vi "Fetch (Unscaled Int16).vi"(0 "VISA resource name":refnum<visa-resource-name>, 1 "Segment Index (0)":i32 format="%.0g", 5 "Measurement Source (1: Channel 1)":i32(ring)=1 items=["Channel 1"=1, "Channel 2"=2, "Channel 3"=3, "Channel 4"=4, "Function 1"=5, "Function 2"=6, "Function 3"=7, "Function 4"=8, "Memory 1"=9, "Memory 2"=10, "Memory 3"=11, "Memory 4"=12], 7 "Number of Samples (1000)":i32=10000 caption="Number of Samples (10000)", 9 "Maximum Time (10000ms)":u32=10000, 11 "error in (no error)":errorcluster, 12 "Offset (0)":i32) -> (4 "VISA resource name out":refnum<visa-resource-name>, 6 "Waveform Information":T1, 8 "Waveform Data":i16[](array[numeric]), 15 "error out":errorcluster)   [LabVIEW 2020, in "Agilent 90000 Series.lvlib"]
doc: "Fetches the unscaled raw word data from instrument. Use this VI under word data format configuration."
uses:
  Agilent 90000 Series.lvlib
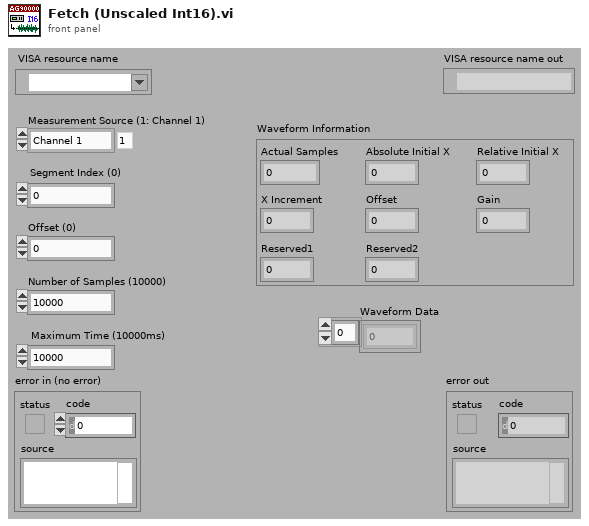
[diagram p1: front panel]
types:
  T1 = cluster{"Actual Samples":i32, "Absolute Initial X":dbl, "Relative Initial X":dbl, "X Increment":dbl, "Offset":dbl, "Gain":dbl, "Reserved1":dbl, "Reserved2":dbl}
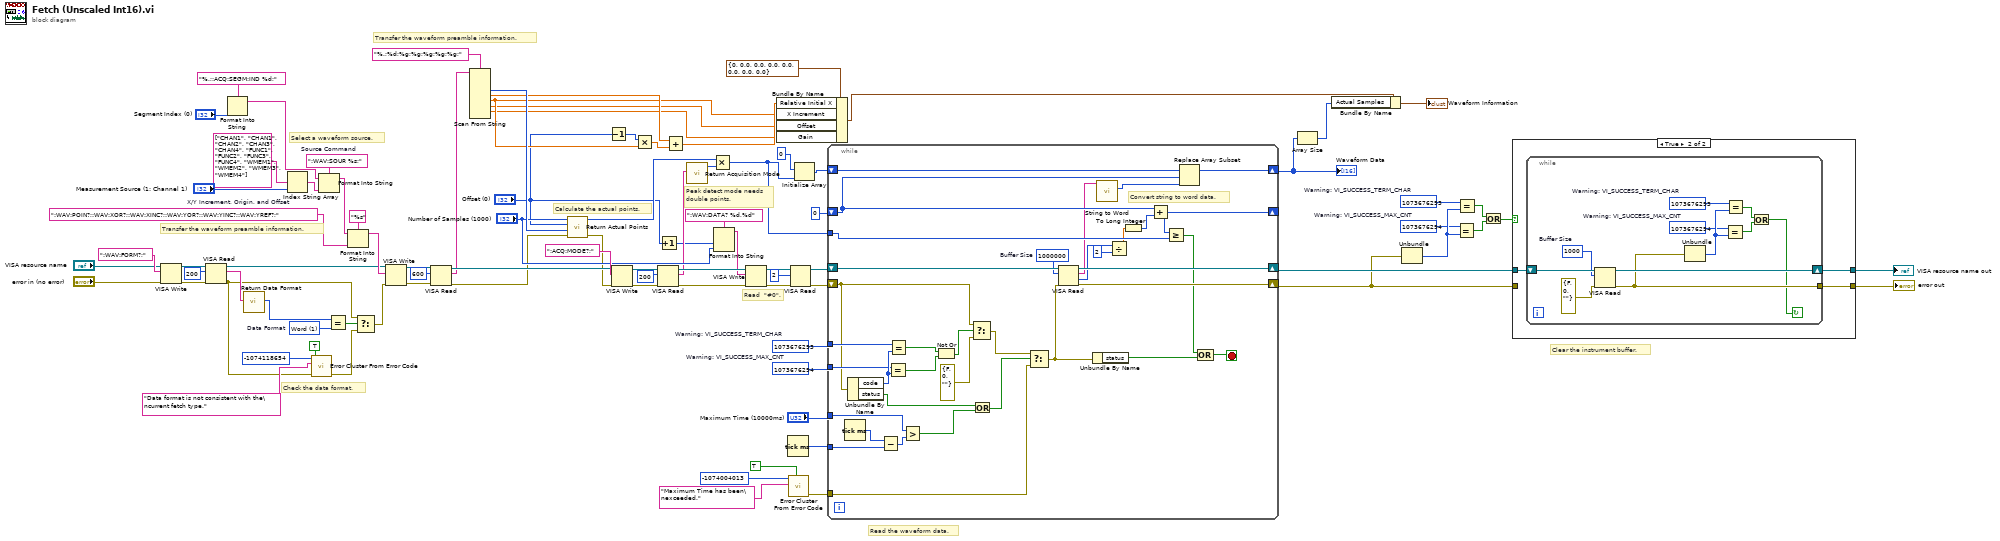
[diagram p0: block diagram]
diagram:
  w18 = u16 1 items=["Byte", "Word", "Others"]  # Data Format
  w74 = 1073676294  # Warning: VI_SUCCESS_MAX_CNT
  w73 = 1073676293  # Warning: VI_SUCCESS_TERM_CHAR
  w67 = 1073676294  # Warning: VI_SUCCESS_MAX_CNT
  w66 = 1073676293  # Warning: VI_SUCCESS_TERM_CHAR
  w87 = ":WAV:SOUR %s;"  # Source Command
  w81 = ":WAV:POIN?;:WAV:XOR?;:WAV:XINC?;:WAV:YOR?;:WAV:YINC?;:WAV:YREF?;"  # X/Y Increment, Origin, and Offset
  # "Transfer the waveform preamble information."
  # "Peak detect mode needs\ndouble points."
  # "Calculate the actual points."
  # "Check the data format."
  # "Read  \"#0\"."
  # "Clear the instrument buffer."
  # "Read the waveform data."
  # "Select a waveform source."
  # "Transfer the waveform preamble information."
  n1 = VISA Write(VISA resource name="VISA resource name", write buffer=":WAV:FORM?;", error in (no error)="error in (no error)") -> (VISA resource name out=w35:refnum<visa-resource-name>, error out=w34:errorcluster)  [unwired: 1 out]
  n2 = VISA Read(VISA resource name=w35, byte count=u32 200, error in (no error)=w34) -> (VISA resource name out=w31:refnum<visa-resource-name>, read buffer=w28:string, error out=w5:errorcluster)  [unwired: 1 out]
  n3 = Format Into String(format string="%.;:ACQ:SEGM:IND %d;", "Segment Index (0)") -> (resulting string=w2:string)  [unwired: 2 in, 1 out]
  n4 = call "Return Data Format.vi"("String In"=w28) -> ("Data Format"=w25:u16)  [unwired: 1 in, 9 out]
  n5 = Index String Array(1:"Measurement Source (1: Channel 1)", 2:string[] ["CHAN1", "CHAN1", "CHAN2", "CHAN3", "CHAN4", "FUNC1", "FUNC2", "FUNC3", "FUNC4", "WMEM1", "WMEM2", "WMEM3", "WMEM4"] ("subarray 2")) -> (0:w82:string)  [unwired: 1 out]
  n6 = call <vilib>:"Error Cluster From Error Code.vi"("show call chain? (False)"=TRUE, "error in (no error)"=w5, "error message (\"\")"="Data format is not consistent with the\ncurrent fetch type." ("error message (\"\")"), "error code (0)"=-1074118654) -> ("error out"=w19:errorcluster)  [unwired: 5 out]
  n7 = Format Into String(format string=w87, initial string=w2, w82) -> (resulting string=w85:string)  [unwired: 1 in, 1 out]
  n8 = Equal?(x=w25, y=w18) -> (x = y?=w24:bool)
  n9 = Format Into String(format string="%s", initial string=w85, w81) -> (resulting string=w84:string)  [unwired: 1 in, 1 out]
  n10 = Select(t=w5, s=w24, f=w19) -> (s? t:f=w23:errorcluster)
  n11 = VISA Write(VISA resource name=w31, write buffer=w84, error in (no error)=w23) -> (VISA resource name out=w90:refnum<visa-resource-name>, error out=w89:errorcluster)  [unwired: 1 out]
  n12 = VISA Read(VISA resource name=w90, byte count=u32 600, error in (no error)=w89) -> (VISA resource name out=w60:refnum<visa-resource-name>, read buffer=w46:string, error out=w9:errorcluster)  [unwired: 1 out]
  n13 = Scan From String(format string="%.;%d;%g;%g;%g;%g;%g;", input string=w46) -> (output 1=w47:i32, output 2=w45:dbl, output 3=w44:dbl, output 4=w13:dbl, output 5=w7:dbl)  [unwired: 2 in, 10 out]
  n14 = call "Return Actual Points.vi"("error in (no error)"=w9, "Total Points (2000)"=w47, "Offset (0)"="Offset (0)", "Number of Samples (1000)"="Number of Samples (1000)") -> ("error out"=w10:errorcluster, "Actual Points"=w41:i32)  [unwired: 6 out]
  n15 = Decrement(x="Offset (0)") -> (x-1=w51:i32)
  n16 = VISA Write(VISA resource name=w60, write buffer=":ACQ:MODE?;", error in (no error)=w10) -> (VISA resource name out=w59:refnum<visa-resource-name>, error out=w58:errorcluster)  [unwired: 1 out]
  n17 = Multiply(x=w51, y=w44) -> (x*y=w50:dbl)
  n18 = VISA Read(VISA resource name=w59, byte count=u32 200, error in (no error)=w58) -> (VISA resource name out=w57:refnum<visa-resource-name>, read buffer=w11:string, error out=w56:errorcluster)  [unwired: 1 out]
  n19 = Increment(x="Offset (0)") -> (x+1=w8:i32)
  n20 = Add(x=w45, y=w50) -> (x+y=w49:dbl)
  n21 = call "Return Acquisition Mode.vi"("Acquisition Mode"=w11) -> ("Multiply Factor"=w12:i32)  [unwired: 10 out]
  n22 = Multiply(x=w41, y=w12) -> (x*y=w40:i32)
  n23 = Format Into String(format string=":WAV:DATA? %d,%d", w8, "Number of Samples (1000)") -> (resulting string=w52:string)  [unwired: 2 in, 1 out]
  n24 = VISA Write(VISA resource name=w57, write buffer=w52, error in (no error)=w56) -> (VISA resource name out=w63:refnum<visa-resource-name>, error out=w62:errorcluster)  [unwired: 1 out]
  n25 = Bundle By Name(cluster=T1 {"Actual Samples"=0, "Absolute Initial X"=0.0, "Relative Initial X"=0.0, "X Increment"=0.0, "Offset"=0.0, "Gain"=0.0, "Reserved1"=0.0, "Reserved2"=0.0} ("Waveform Information"), "Relative Initial X"=w49, "X Increment"=w44, "Offset"=w13, "Gain"=w7) -> (w16:T1)
  n26 = Tick Count (ms)() -> (millisecond timer value=w72:u32)
  n27 = call <vilib>:"Error Cluster From Error Code.vi"("show call chain? (False)"=TRUE, "error message (\"\")"="Maximum Time has been\nexceeded." ("error message (\"\")"), "error code (0)"=-1074004013) -> ("error out"=w6:errorcluster)  [unwired: 1 in, 5 out]
  n28 = VISA Read(VISA resource name=w63, byte count=u32 2, error in (no error)=w62) -> (VISA resource name out=w42:refnum<visa-resource-name>, error out=w43:errorcluster)  [unwired: 2 out]
  n29 = Initialize Array(i16 0 ("element"), w40) -> (w27:i16[])
  n30 = while {
    shift-right: [w121] -> w79
    shift-left: w43 -> [w109]
    shift-right: [w126] -> w80
    shift-left: w42 -> [w125]
    shift-right: [w122] -> w1
    shift-left: w27 -> [w123]
    shift-right: [w119] -> _
    shift-left: 0 ("index") -> [w120]
    tunnel: w40 -> [w118]
    tunnel: w66 -> [w111]
    tunnel: w67 -> [w110]
    tunnel: "Maximum Time (10000ms)" -> [w106]
    tunnel: w72 -> [w105]
    tunnel: w6 -> [w100]
    stop <- w97 stop-if-true
    w124 = u32 1000000  # Buffer Size
    # "Convert string to word data."
    n31 = Tick Count (ms)() -> (millisecond timer value=w107:u32)
    n32 = Unbundle By Name(w109) -> ("code"=w112:i32, "status"=w104:bool)
    n33 = Subtract(x=w107, y=w105) -> (x-y=w108:u32)
    n34 = Equal?(x=w110, y=w112) -> (x = y?=w115:bool)
    n35 = Equal?(x=w111, y=w112) -> (x = y?=w116:bool)
    n36 = Greater?(x=w106, y=w108) -> (0:w103:bool)
    n37 = Not Or(1:w115, 2:w116) -> (0:w114:bool)
    n38 = Select(t=w109, s=w114, f=errorcluster {"status"=FALSE, "code"=0, "source"=""} ("error in (no error)")) -> (s? t:f=w102:errorcluster)
    n39 = Or(x=w104, y=w103) -> (x .or. y?=w101:bool)
    n40 = Select(t=w102, s=w101, f=w100) -> (s? t:f=w99:errorcluster)
    n41 = VISA Read(VISA resource name=w125, byte count=w124, error in (no error)=w99) -> (VISA resource name out=w126:refnum<visa-resource-name>, read buffer=w91:string, return count=w95:u32, error out=w121:errorcluster)
    n42 = Unbundle By Name(w99) -> ("status"=w98:bool)
    n43 = call "String to Word.vi"("String"=w91) -> ("Int16 Data"=w92:i16[])  [unwired: 1 in, 9 out]
    n44 = Divide(x=w95, y=u32 2) -> (x/y=w96:dbl)
    n45 = To Long Integer(number=w96) -> (32bit integer=w93:i32)
    n46 = Add(x=w120, y=w93) -> (x+y=w119:i32)
    n47 = Greater Or Equal?(x=w119, y=w118) -> (x >= y?=w117:bool)
    n48 = Replace Array Subset(array=w123, new element=w92, index=w120) -> (w122:i16[])
    n49 = Compound Arithmetic op=OR(w117, w98) -> (w97:bool)
  }
  "Waveform Data" <- w1
  n50 = Array Size(array=w1) -> (size(s)=w15:i32)
  n51 = Bundle By Name(cluster=w16, "Actual Samples"=w15) -> (→"Waveform Information":T1)
  n52 = Unbundle(w79) -> ("code"=w75:i32)  [unwired: 2 out]
  n53 = Equal?(x=w74, y=w75) -> (x = y?=w77:bool)
  n54 = Equal?(x=w73, y=w75) -> (x = y?=w78:bool)
  n55 = Or(x=w78, y=w77) -> (x .or. y?=w76:bool)
  n56 = case shown="True" w76 {
    tunnel: w80 -> [w128 w131]
    tunnel: w79 -> [w127 _]
    tunnel: [w128 w130] -> w38
    tunnel: [w127 w129] -> w37
    frame False {
    }
    frame True {
      n57 = while {
        shift-right: [w141] -> w130
        shift-left: w131 -> [w142]
        tunnel: [w134] -> w129
        stop <- w133 continue-if-true
        w136 = 1073676294  # Warning: VI_SUCCESS_MAX_CNT
        w135 = 1073676293  # Warning: VI_SUCCESS_TERM_CHAR
        w140 = u32 1000  # Buffer Size
        n58 = VISA Read(VISA resource name=w142, byte count=w140, error in (no error)=errorcluster {"status"=FALSE, "code"=0, "source"=""}) -> (VISA resource name out=w141:refnum<visa-resource-name>, error out=w134:errorcluster)  [unwired: 2 out]
        n59 = Unbundle(w134) -> ("code"=w137:i32)  [unwired: 2 out]
        n60 = Equal?(x=w136, y=w137) -> (x = y?=w138:bool)
        n61 = Equal?(x=w135, y=w137) -> (x = y?=w139:bool)
        n62 = Or(x=w139, y=w138) -> (x .or. y?=w133:bool)
      }
    }
  }
  "error out" <- w37
  "VISA resource name out" <- w38
